vi "ATM.vi"() -> ()   [LabVIEW 2024]
doc: "This VI Simulates the operation of an ATM. It has option to simulate the card, informs the user via the ATM message. It has 6 buttons/ menus that the user can use to select the action he/she wants to perform"
uses:
  Next State.ctl
  Previous State.ctl
  <vilib>/Utility/file.llb/Read Delimited Spreadsheet (string).vi
  <vilib>/Utility/file.llb/Write Delimited Spreadsheet (string).vi
panel:
  in  "Enter":bool
  in  "User Input":string
  in  "Right Buttons\nButtons":T1
  out "Right Menu":T2
  in  "Left Buttons":T1
  out "Left Menu":T2
  in  "Card Simulator":bool
  out "ATM Messages":string
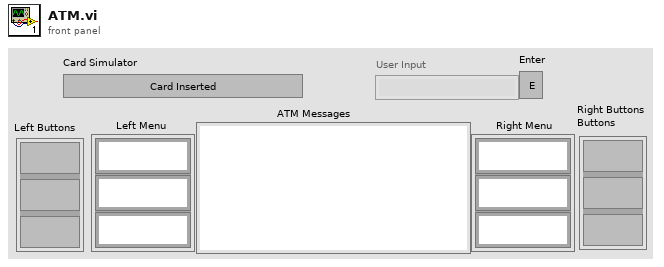
[diagram p1: front panel]
types:
  T1 = cluster{"Func Button":bool, "Func Button 2":bool, "Func Button 3":bool}
  T2 = cluster{"RFS String":string, "RFS String 2":string, "RFS String 3":string}
  T3 = typedef "Previous State.ctl" = enum16{"Start", "Withdraw", "Deposit", "Card Inserted"}
  T4 = cluster{"appended path":path, "Previous State":T3, "User Input":string, "File data":string[][], "Account Number Index":i32}
  T5 = cluster{"User Input":refnum<vi>, "Left Buttons":refnum<vi>, "Right Buttons\nButtons":refnum<vi>, "Enter":refnum<vi>, "Card Simulator":refnum<vi>}
  T6 = typedef "Next State.ctl" = enum16{"Start/Run", "Wait for Event", "Session Terminate", "Exit"}
  T7 = cluster{"Left Menu":cluster{"RFS String":string, "RFS String 2":string, "RFS String 3":string}, "ATM Messages":string, "Right Menu":cluster{"RFS String":string, "RFS String 2":string, "RFS String 3":string}}
  T8 = enum16{"Balance Inquiry", "Withdrawal Failed", "Withdrawal Complete", "Withdrawal", "Deposit Complete", "Deposit", "Session Terminate", "Account Verification Failed", "Main Menu", "Welcome Message"}
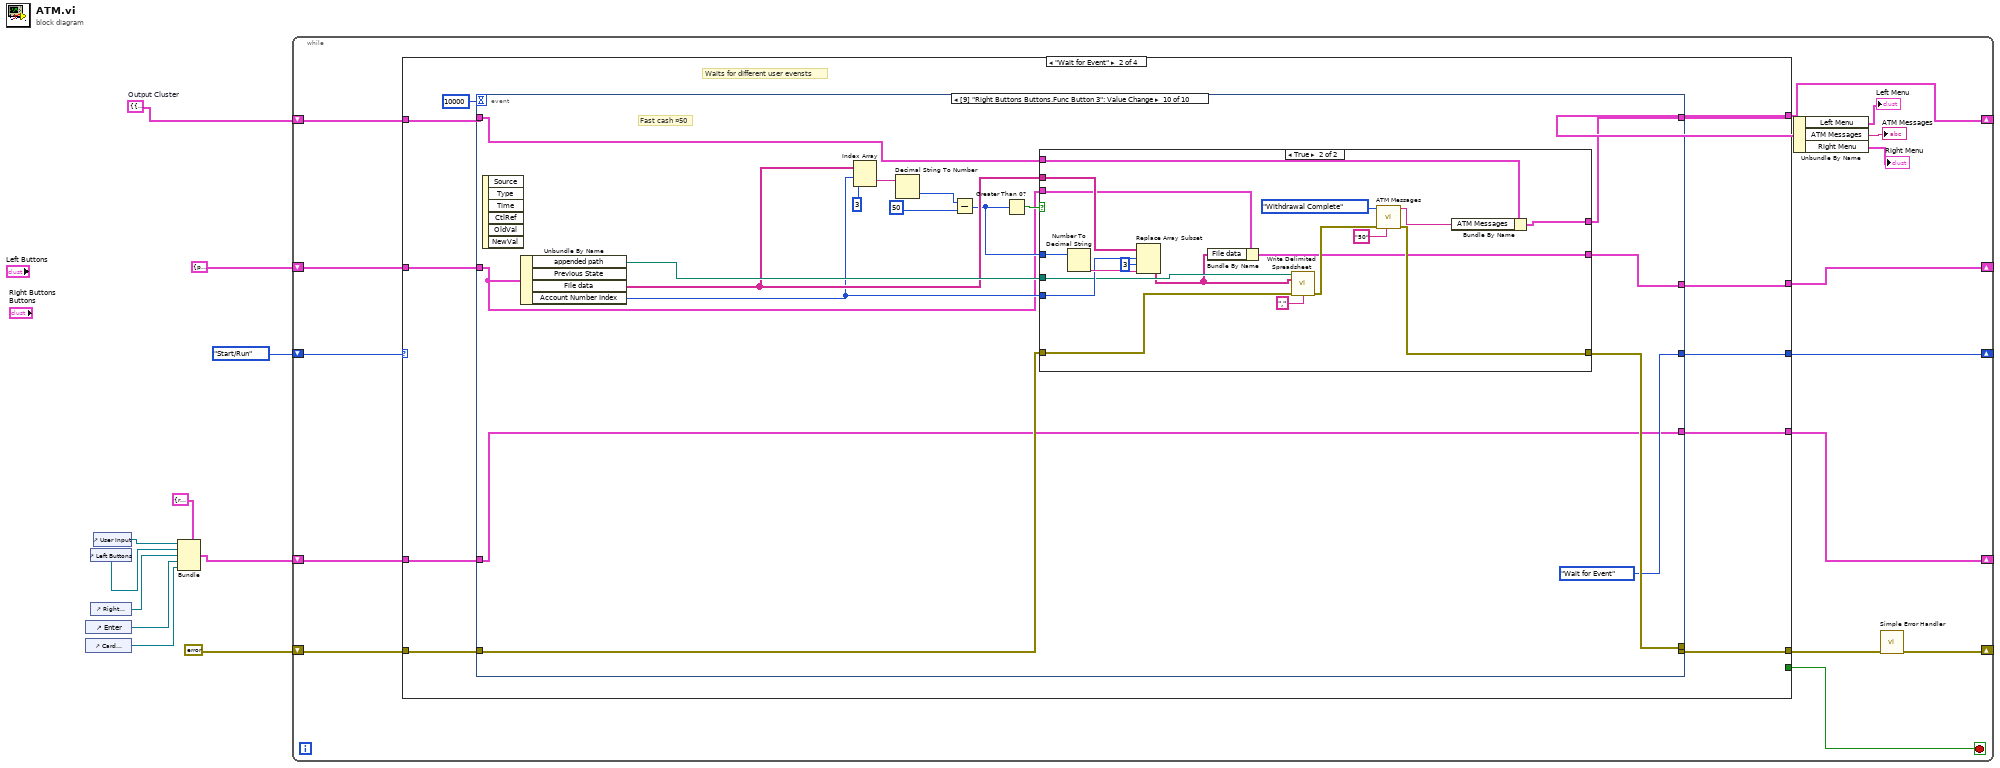
[diagram p0: block diagram]
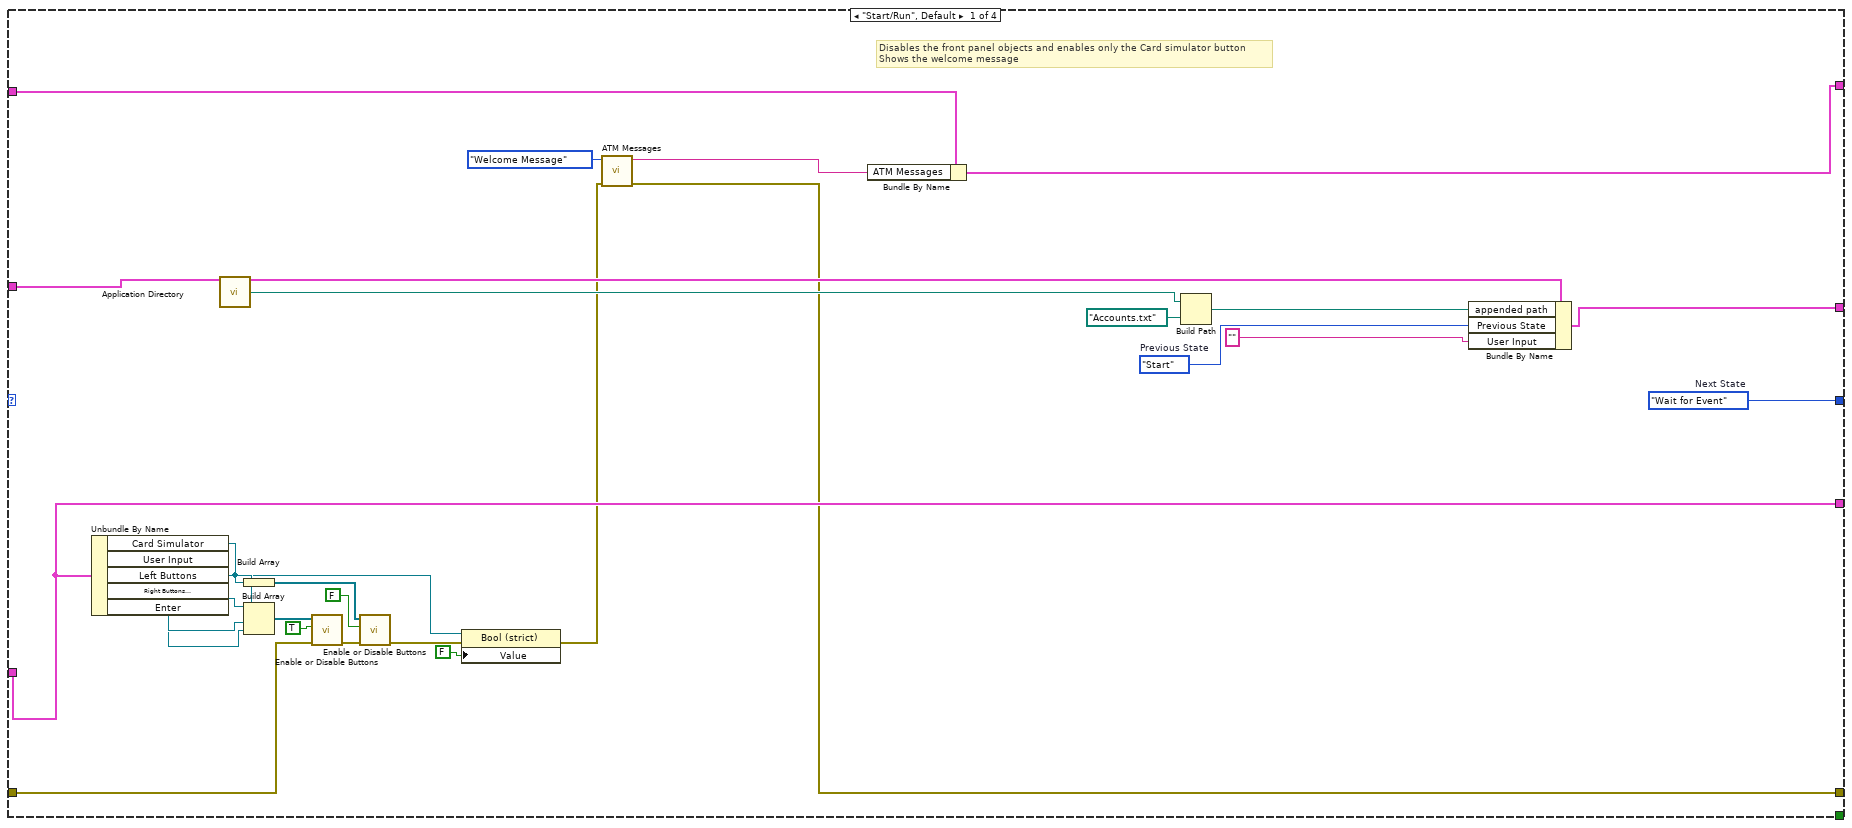
[diagram p2: hidden frame]
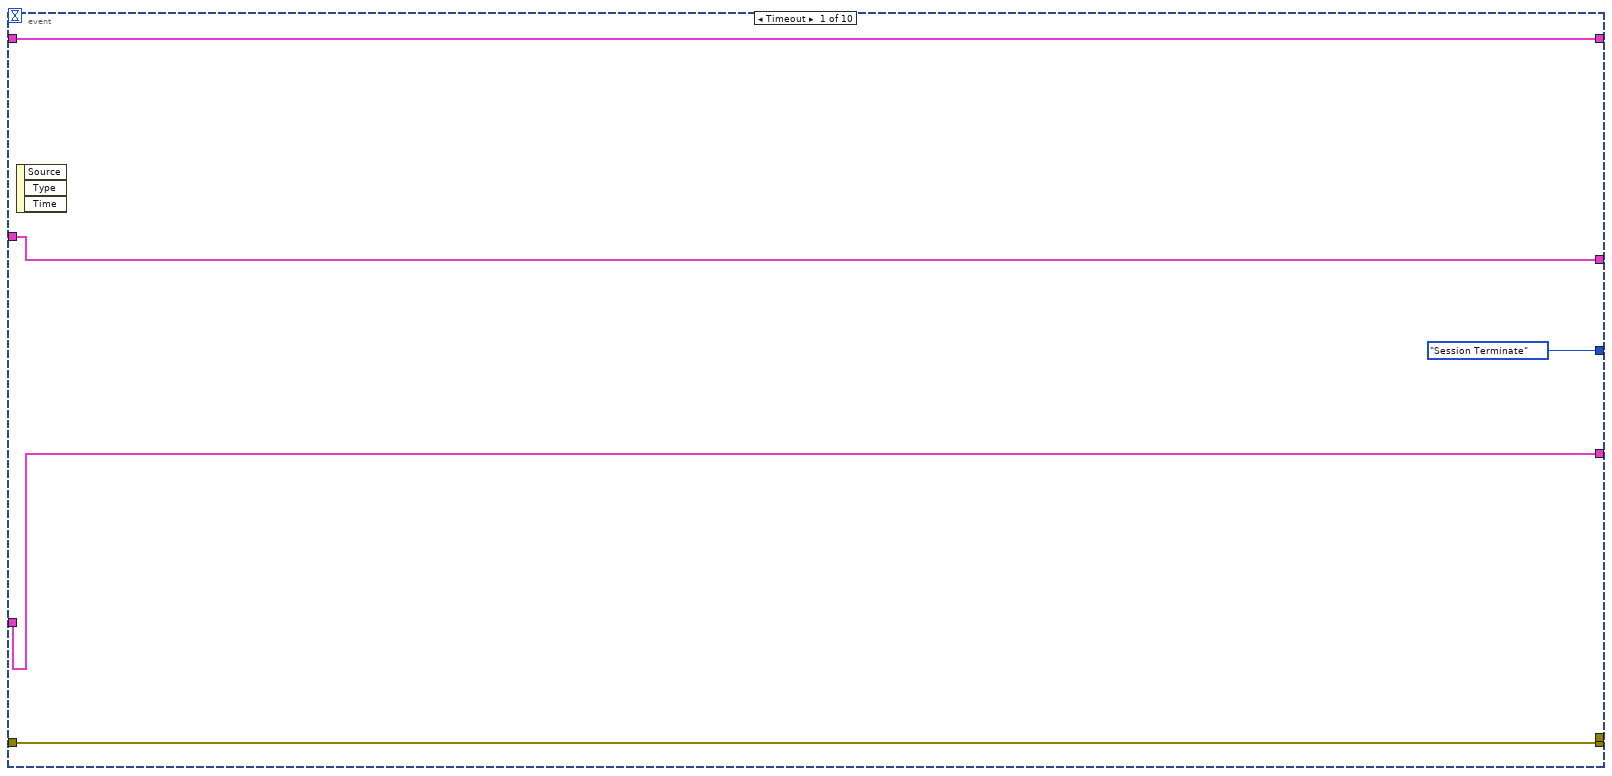
[diagram p3: hidden frame]
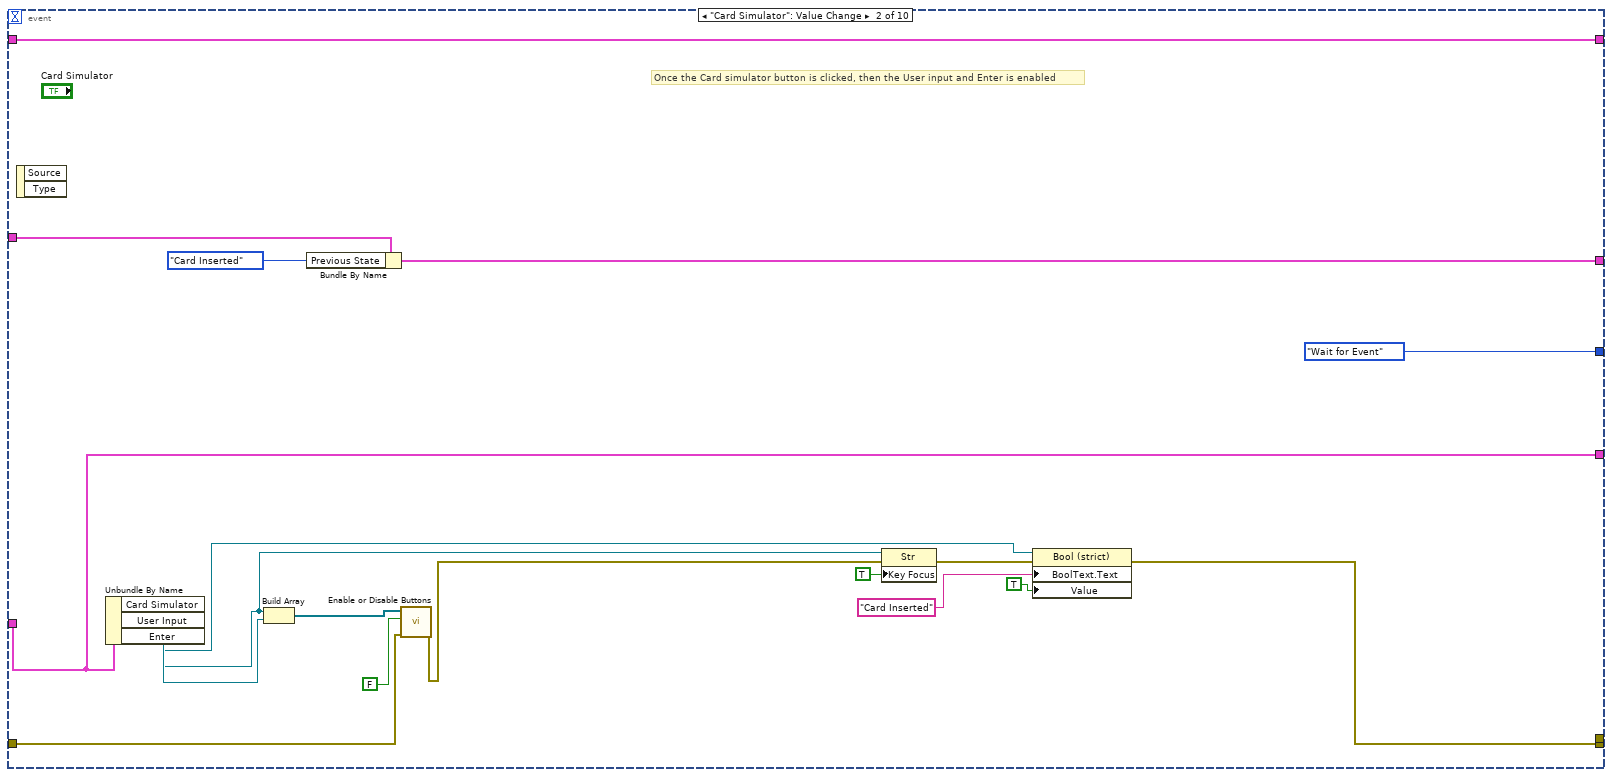
[diagram p4: hidden frame]
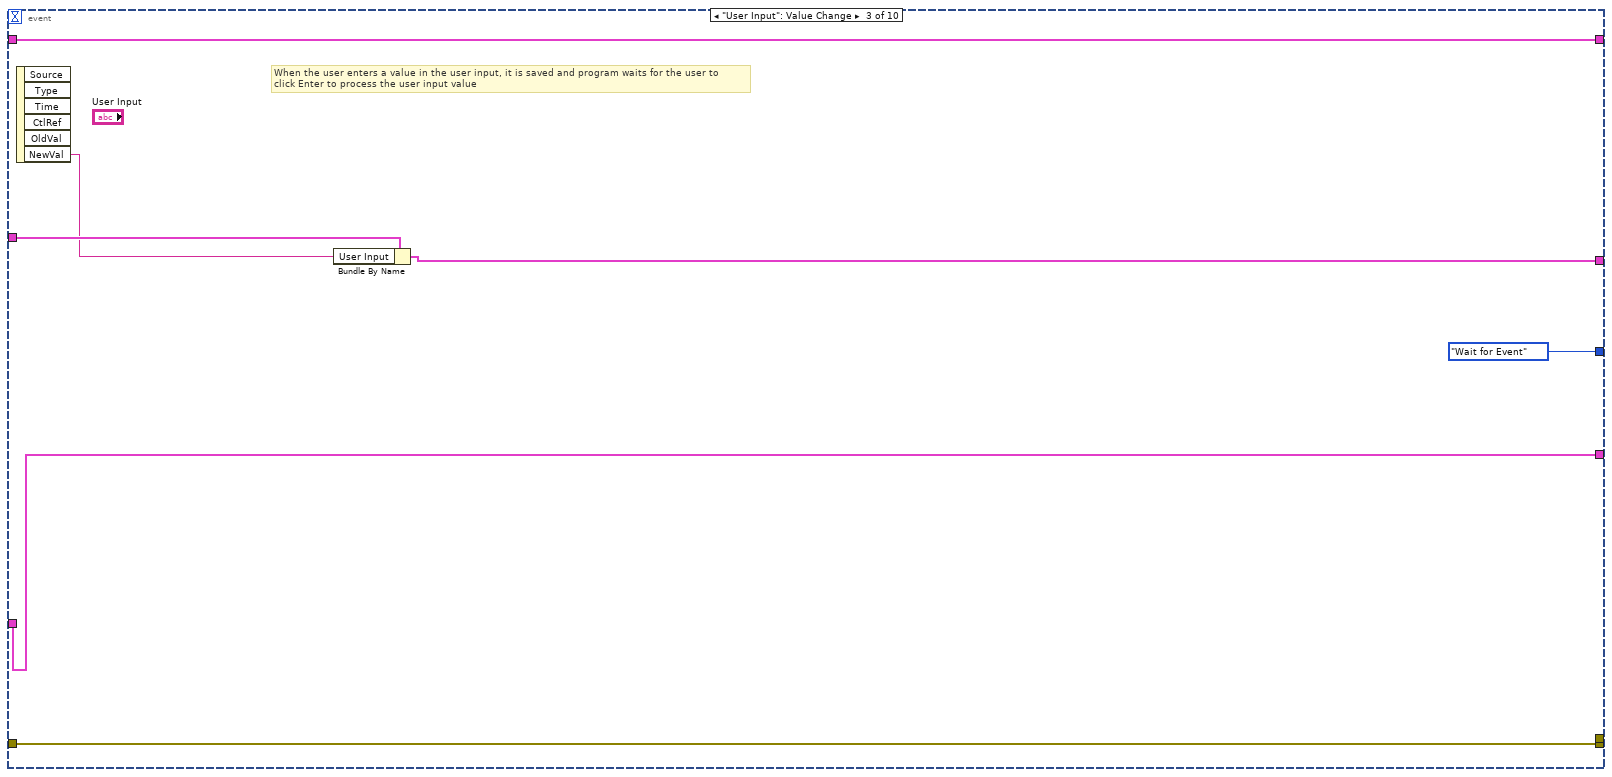
[diagram p5: hidden frame]
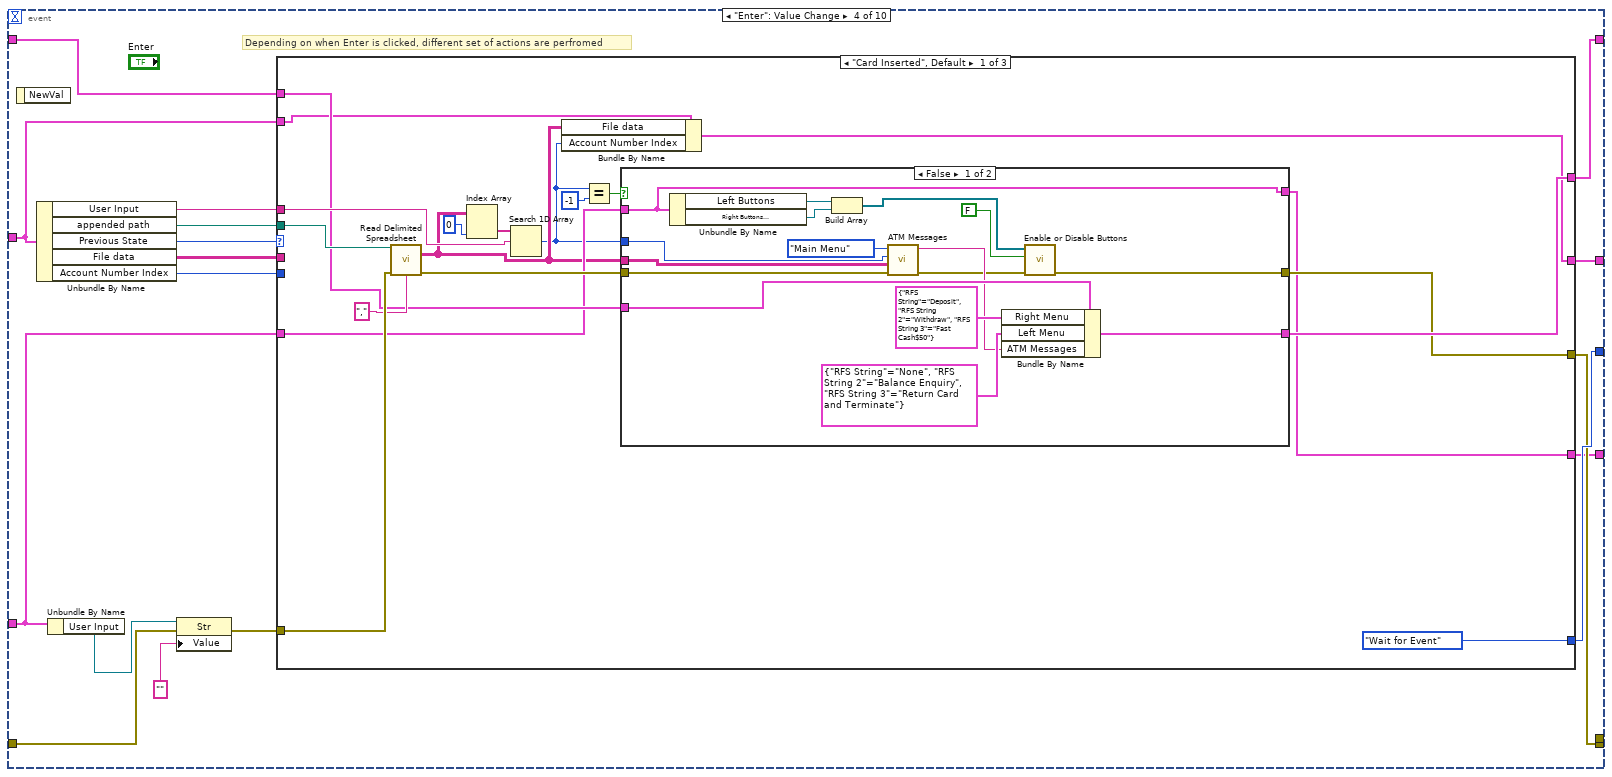
[diagram p6: hidden frame]
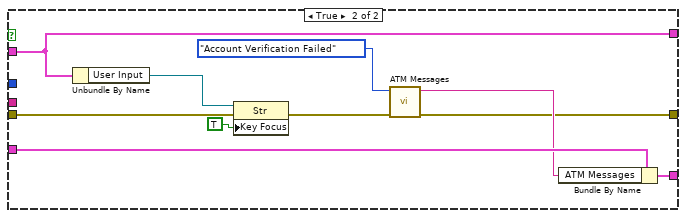
[diagram p7: hidden frame]
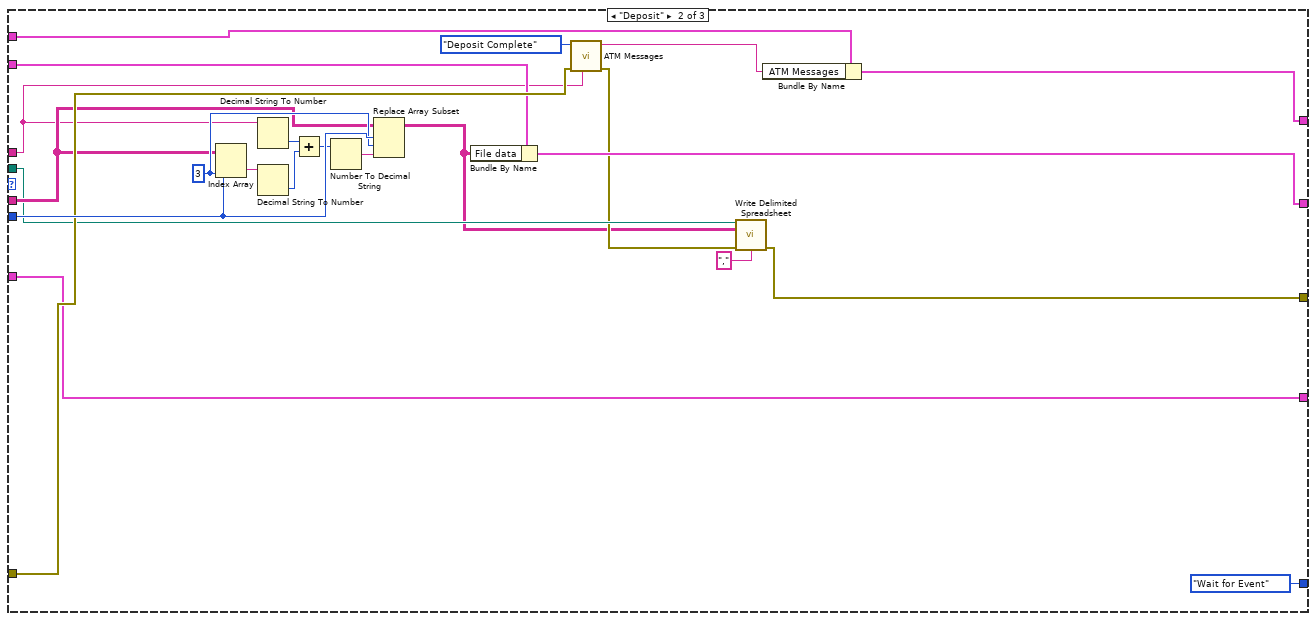
[diagram p8: hidden frame]
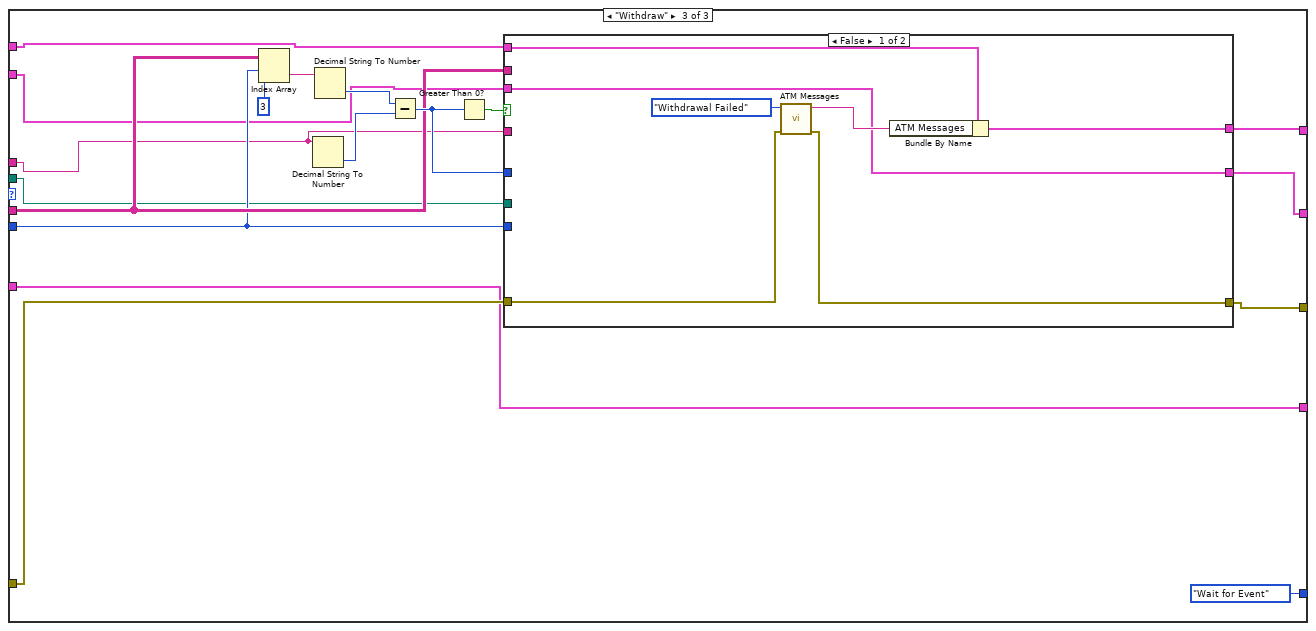
[diagram p9: hidden frame]
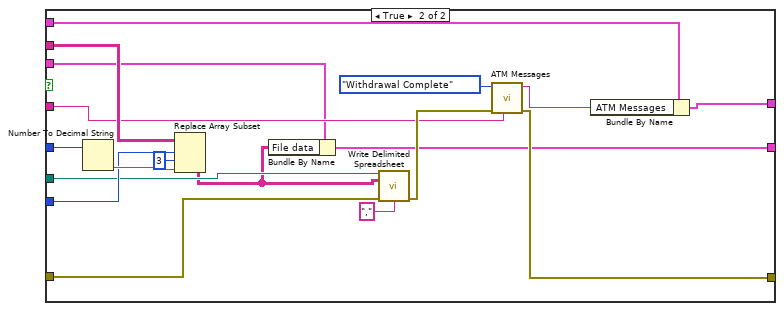
[diagram p10: hidden frame]
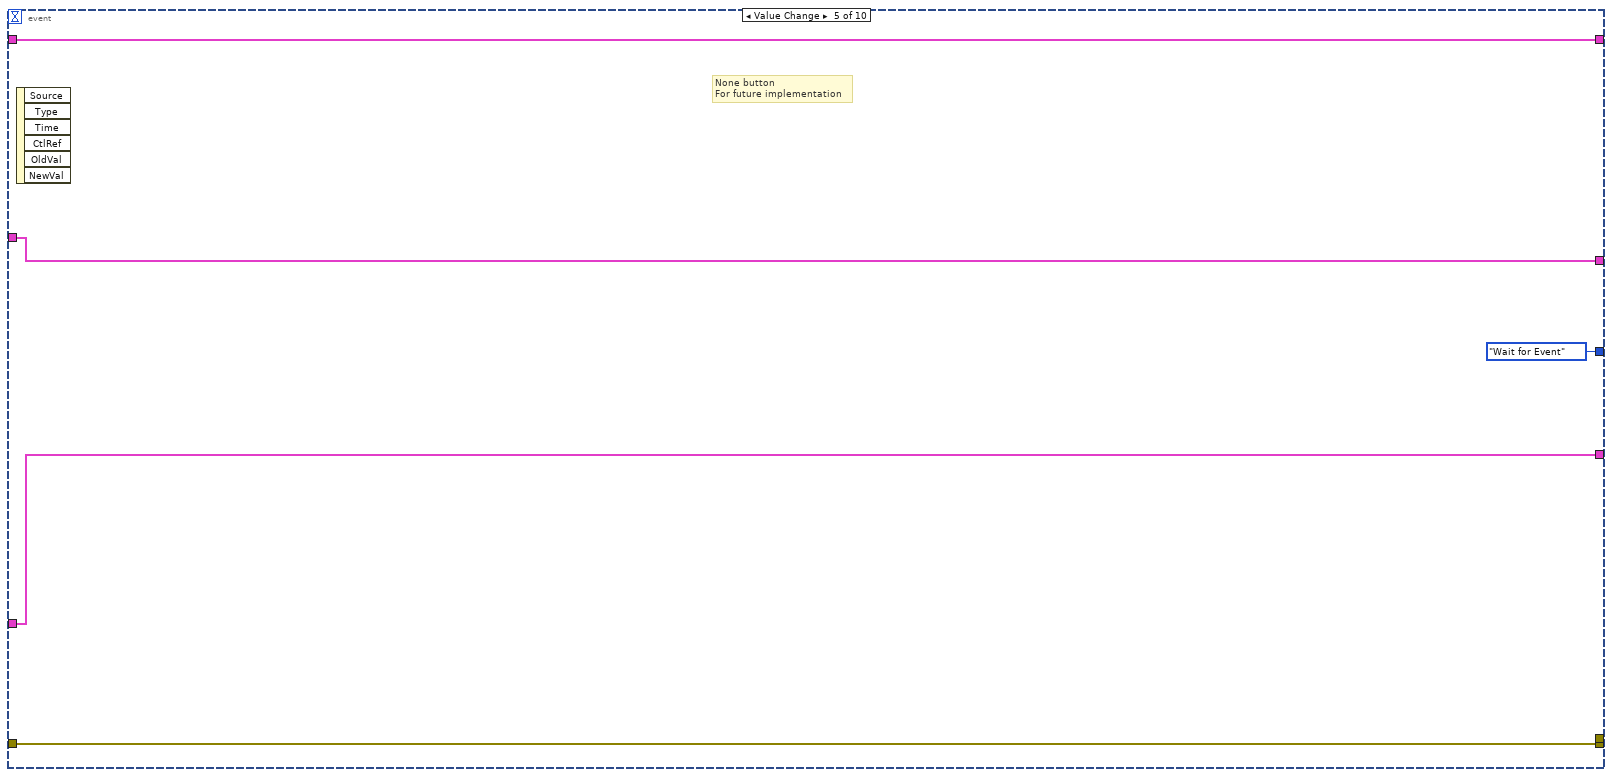
[diagram p11: hidden frame]
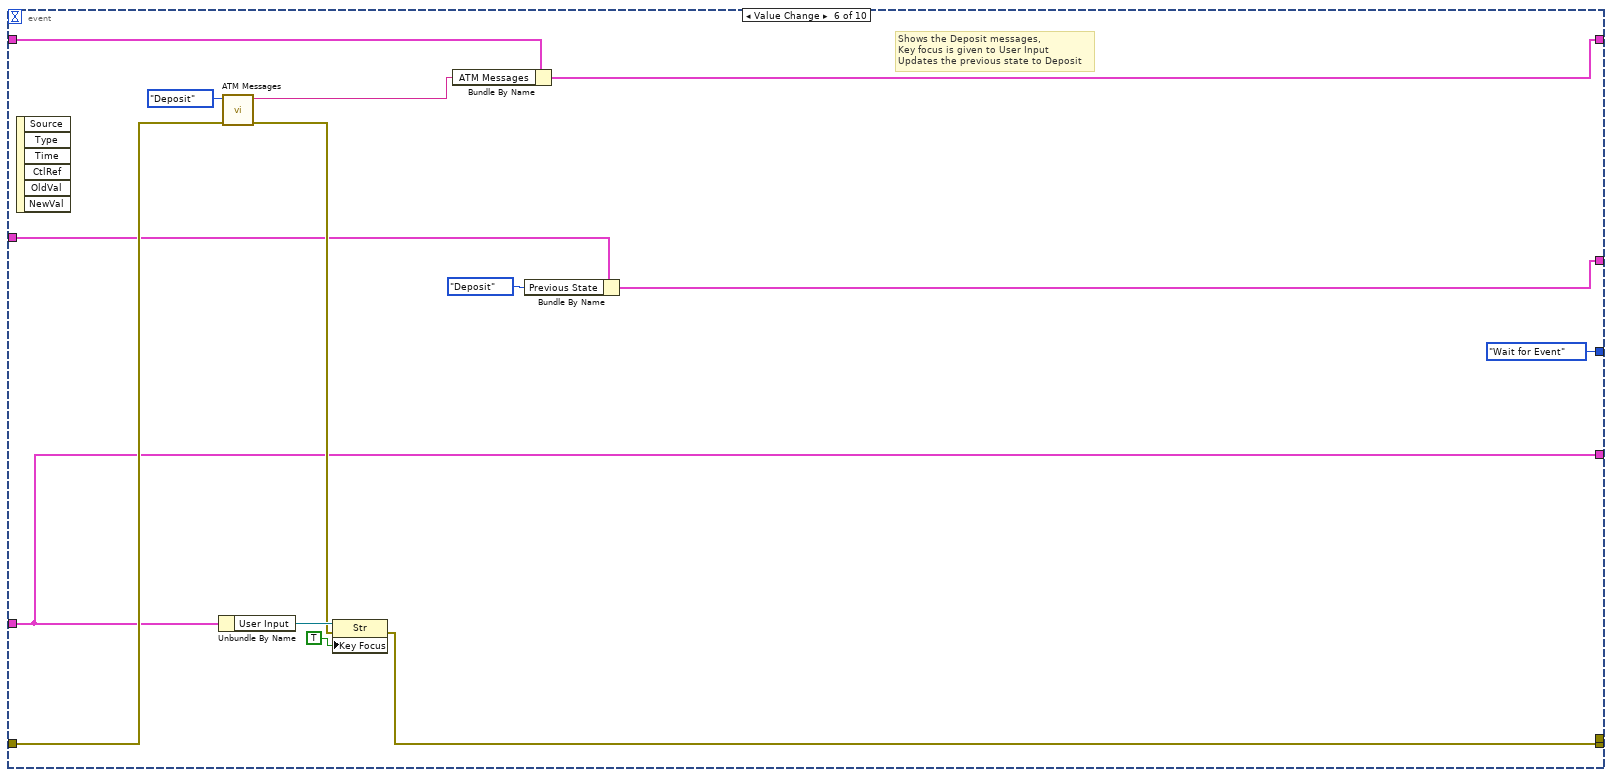
[diagram p12: hidden frame]
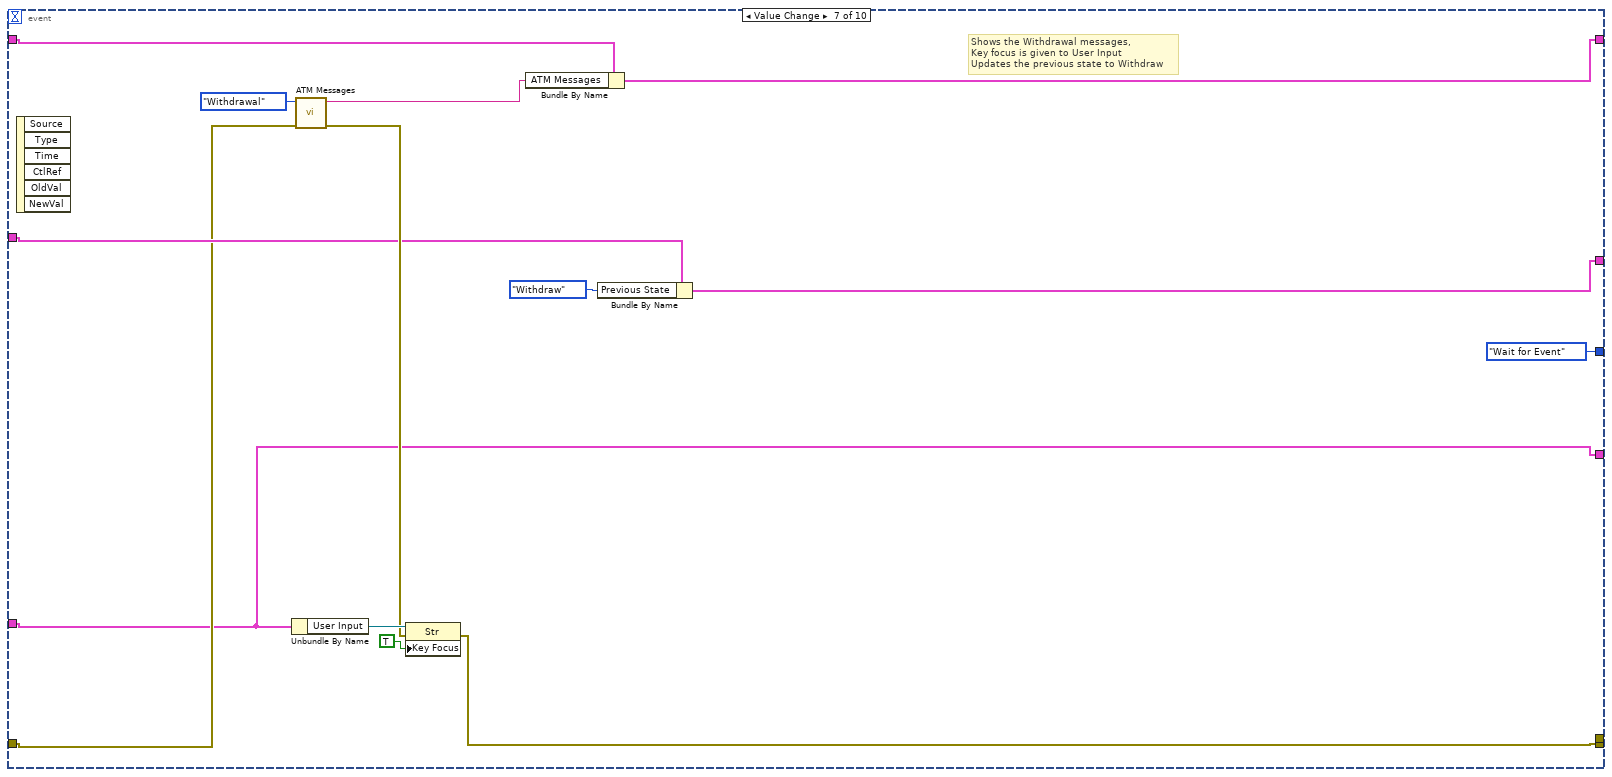
[diagram p13: hidden frame]
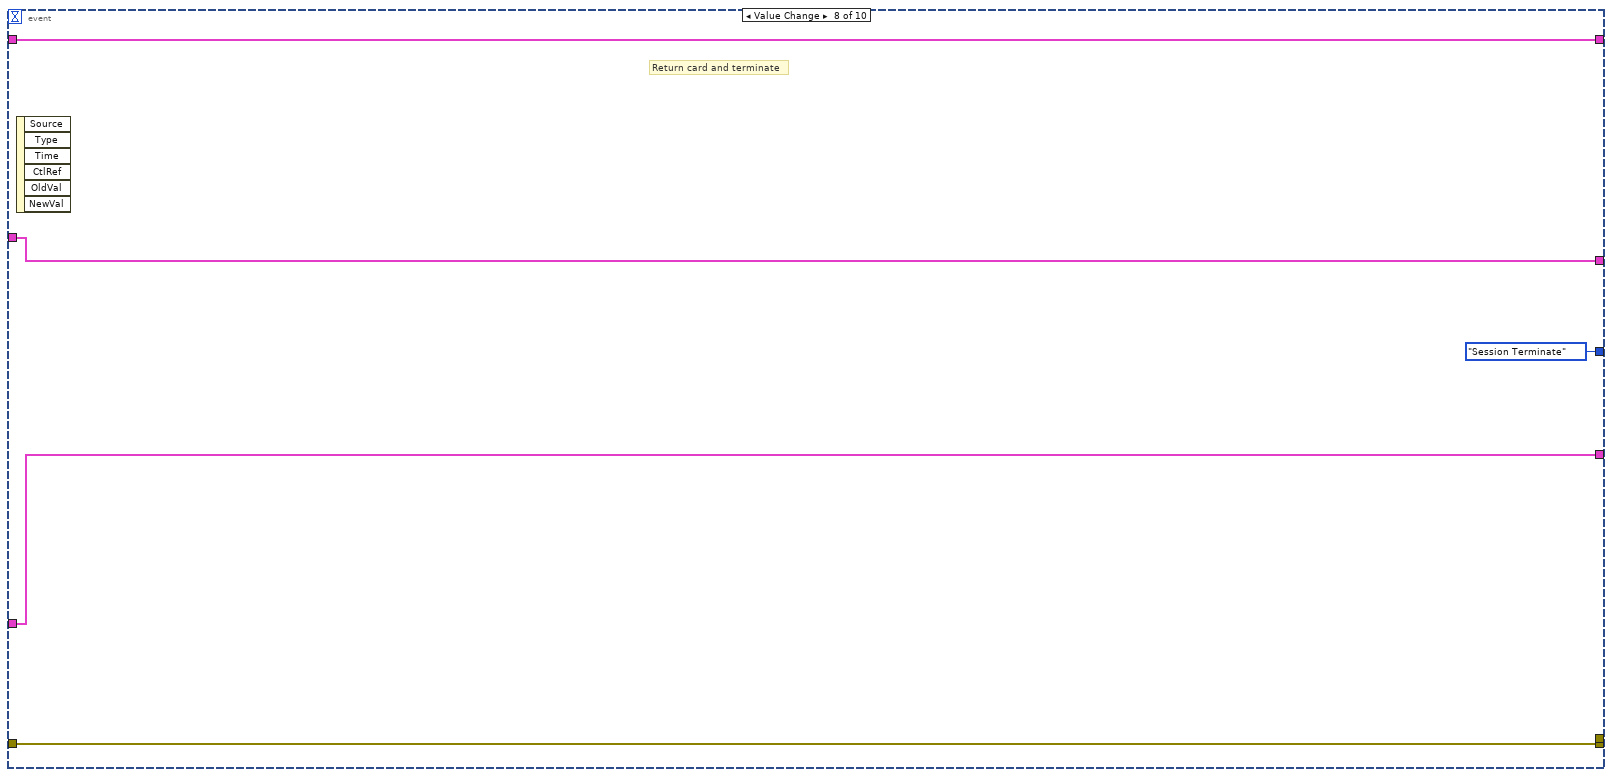
[diagram p14: hidden frame]
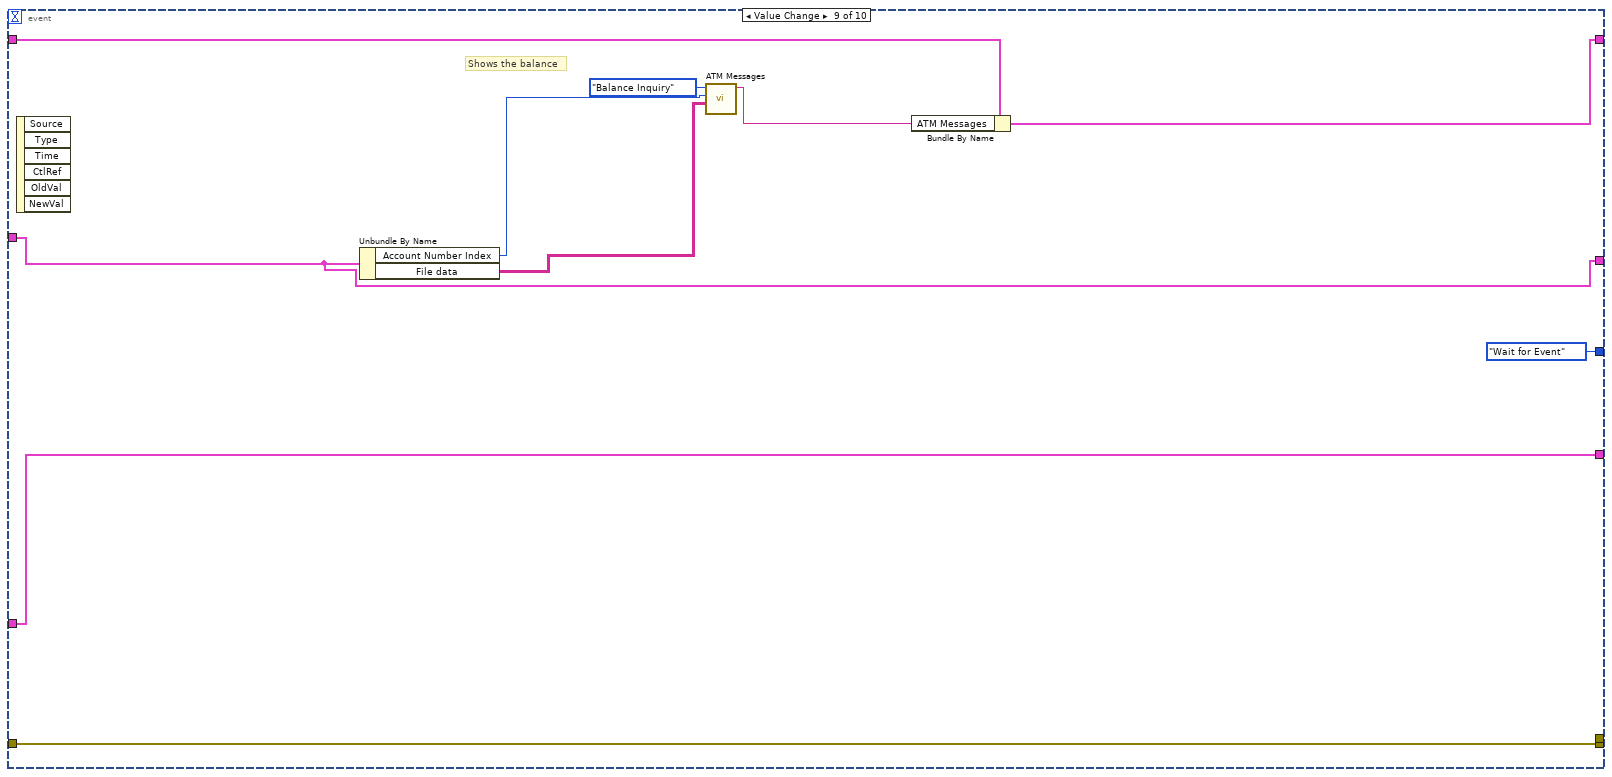
[diagram p15: hidden frame]
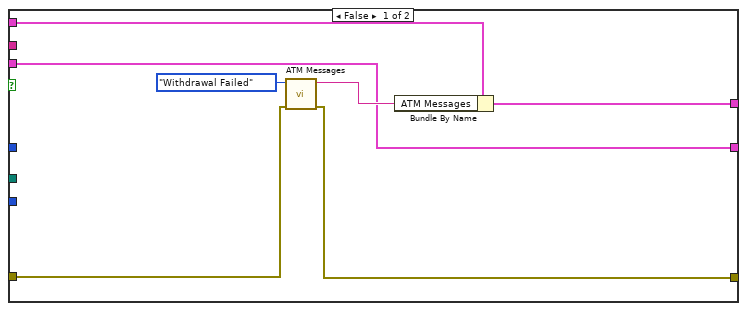
[diagram p16: hidden frame]
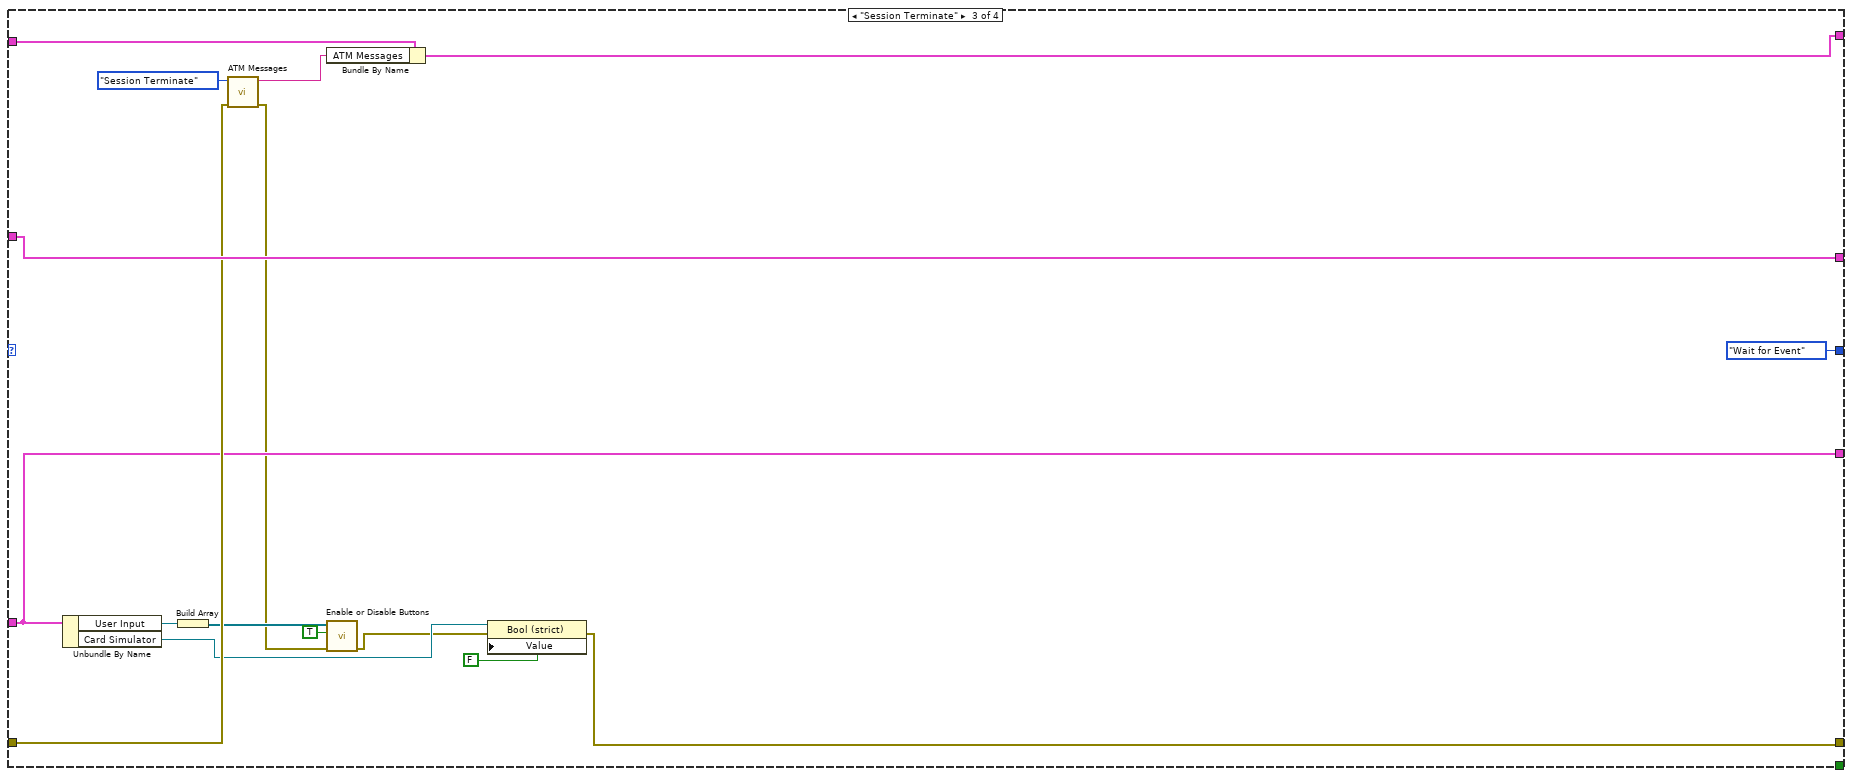
[diagram p17: hidden frame]
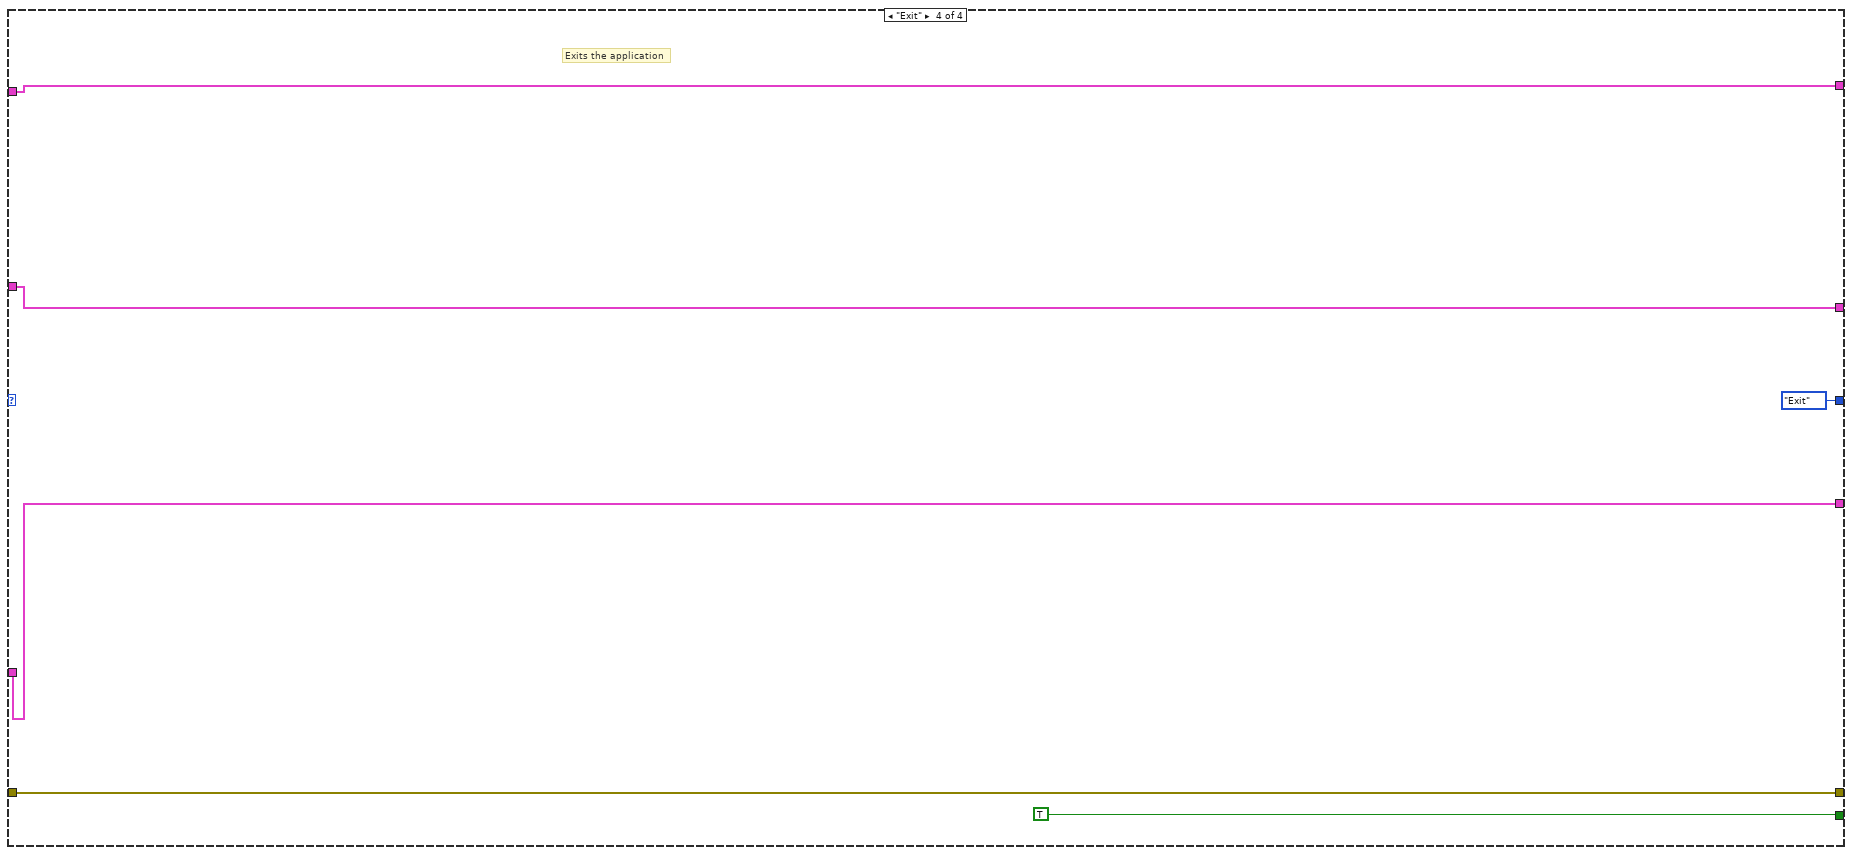
[diagram p18: hidden frame]
diagram:
  w11 = T7 {"Left Menu"={"RFS String"="", "RFS String 2"="", "RFS String 3"=""}, "ATM Messages"="", "Right Menu"={"RFS String"="", "RFS String 2"="", "RFS String 3"=""}}  # Output Cluster
  n1 = control-ref of="Enter"() -> (w6:refnum<vi>)
  n2 = control-ref of="Card Simulator"() -> (w5:refnum<vi>)
  n3 = control-ref of="Left Buttons"() -> (w8:refnum<vi>)
  n4 = control-ref of="Right Buttons\nButtons"() -> (w7:refnum<vi>)
  n5 = control-ref of="User Input"() -> (w9:refnum<vi>)
  n6 = Bundle(cluster=T5 {"User Input"=refnum, "Left Buttons"=refnum, "Right Buttons\nButtons"=refnum, "Enter"=refnum, "Card Simulator"=refnum}, "User Input"=w9, "Left Buttons"=w8, "Right Buttons\nButtons"=w7, "Enter"=w6, "Card Simulator"=w5) -> (w3:T5)
  n7 = while {
    shift-right: [w22] -> _
    shift-left: w11 -> [w26]
    shift-right: [w17] -> _
    shift-left: w3 -> [w19]
    shift-right: [w12] -> _
    shift-left: errorcluster {"status"=FALSE, "code"=0, "source"=""} ("error out") -> [w18]
    shift-right: [w16] -> _
    shift-left: Next_State."Start/Run" -> [w21]
    shift-right: [w14] -> _
    shift-left: T4 {"appended path"=path "", "Previous State"=enum."Withdraw", "User Input"="", "File data"=[], "Account Number Index"=0} ("Data") -> [w15]
    stop <- w20 stop-if-true
    n8 = case shown="\"Wait for Event\"" w21 {
      tunnel: w26 -> [w42 w61 w328 w333]
      tunnel: [w41 w55 w327 w333] -> w22
      tunnel: [_ _ _ TRUE] -> w20
      tunnel: w19 -> [w45 w63 w321 w331]
      tunnel: w18 -> [w48 w62 w322 w329]
      tunnel: [w45 w56 w321 w331] -> w17
      tunnel: [w40 w57 Next_State."Wait for Event" ("Next State") Next_State."Exit" ("Next State")] -> w16
      tunnel: w15 -> [w39 w59 w325 w332]
      tunnel: [w35 w58 w325 w332] -> w14
      tunnel: [w27 w60 w314 w329] -> w13
      frame "Start/Run", Default {
        w40 = Next_State."Wait for Event"  # Next State
        w37 = Previous_State."Start"  # Previous State
        # "Disables the front panel objects and enables only the Card simulator button\nShows the welcome message"
        n9 = Unbundle By Name(w45) -> ("Card Simulator"=w33:refnum<vi>, "User Input"=w54:refnum<vi>, "Left Buttons"=w53:refnum<vi>, "Right Buttons\nButtons"=w52:refnum<vi>, "Enter"=w51:refnum<vi>)
        n10 = call <vilib>:"Application Directory.vi"() -> ("Application Directory"=w44:path)
        n11 = Build Array(w33) -> (w47:refnum<vi>[])
        n12 = Build Array(w54, w53, w52, w51) -> (w50:refnum<vi>[])
        n13 = call "Enable or Disable Buttons.vi"("Error In"=w48, "Disable?"=TRUE, "Refnum array"=w50) -> ("Error Out"=w34:errorcluster)  [unwired: 7 in, 1 out]
        n14 = call "Enable or Disable Buttons.vi"("Error In"=w34, "Disable?"=FALSE, "Refnum array"=w47) -> ("Error Out"=w31:errorcluster)  [unwired: 7 in, 1 out]
        n15 = property class="Bool (strict)"(reference=w33, error in=w31, "Value"=FALSE) -> (error out=w28:errorcluster)  [unwired: 1 out]
        n16 = call "ATM Messages.vi"("Error In"=w28, "Atm Message"=T8."Welcome Message") -> ("error Out"=w27:errorcluster, "ATM Messages"=w29:string)  [unwired: 8 in]
        n17 = Bundle By Name(cluster=w42, "ATM Messages"=w29) -> (w41:T7)
        n18 = Build Path(base path=w44, name or relative path=path "Accounts.txt") -> (appended path=w38:path)
        n19 = Bundle By Name(cluster=w39, "appended path"=w38, "Previous State"=w37, "User Input"="") -> (w35:T4)
      }
      frame "Wait for Event" {
        # "Waits for different user evensts"
        n20 = event shown="[9] \"Right Buttons Buttons.Func Button 3\": Value Change" {
          selector: _ -> [_ _ _ _ _ _ _ _ _ _]
          dyn-events: _ -> [_ _ _ _ _ _ _ _ _ _]
          timeout: 10000 -> [_ _ _ _ _ _ _ _ _ _]
          tunnel: w63 -> [w67 w75 w91 w100 w226 w228 w242 w259 w263 w272]
          tunnel: w62 -> [w66 w84 w92 w110 w227 w235 w247 w260 w264 w278]
          tunnel: w61 -> [w69 w80 w89 w104 w223 w240 w249 w256 w267 w277]
          tunnel: [w69 w80 w89 w103 w223 w238 w243 w256 w265 w271] -> w55
          tunnel: [w66 w71 w92 w101 w227 w233 w246 w260 w264 _] -> w60
          tunnel: w59 -> [w68 w79 w94 w99 w224 w232 w248 w257 w262 w276]
          tunnel: [w68 w77 w93 w97 w224 w230 w244 w257 w262 w275] -> w58
          tunnel: [Next_State."Session Terminate" ("Next State") Next_State."Wait for Event" ("Next State") Next_State."Wait for Event" ("Next State") w105 Next_State."Wait for Event" ("Next State") Next_State."Wait for Event" ("Next State") Next_State."Wait for Event" ("Next State") Next_State."Session Terminate" ("Next State") Next_State."Wait for Event" ("Next State") Next_State."Wait for Event" ("Next State")] -> w57
          tunnel: [w67 w75 w91 w98 w226 w228 w242 w259 w263 w272] -> w56
          tunnel: [_ _ _ _ _ _ _ _ _ w274] -> _
          event Timeout {
            n21 = event-data() -> ()  [unwired: 1 in, 3 out]
          }
          event "Card Simulator": Value Change {
            # "Once the Card simulator button is clicked, then the User input and Enter is enabled"
            n22 = event-data() -> ()  [unwired: 1 in, 2 out]
            n23 = Unbundle By Name(w75) -> ("Card Simulator"=w74:refnum<vi>, "User Input"=w83:refnum<vi>, "Enter"=w87:refnum<vi>)
            n24 = Build Array(w83, w87) -> (w86:refnum<vi>[])
            n25 = Bundle By Name(cluster=w79, "Previous State"=Previous_State."Card Inserted") -> (w77:T4)
            n26 = call "Enable or Disable Buttons.vi"("Error In"=w84, "Disable?"=FALSE, "Refnum array"=w86) -> ("Error Out"=w82:errorcluster)  [unwired: 7 in, 1 out]
            n27 = property class="Str"(reference=w83, error in=w82, "Key Focus"=TRUE) -> (error out=w72:errorcluster)  [unwired: 1 out]
            n28 = property class="Bool (strict)"(reference=w74, error in=w72, "BoolText.Text"="Card Inserted" ("Boolean Text.Text"), "Value"=TRUE) -> (error out=w71:errorcluster)  [unwired: 1 out]
          }
          event "User Input": Value Change {
            # "When the user enters a value in the user input, it is saved and program waits for the user to \nclick Enter to process the user input value"
            n29 = event-data() -> ("NewVal"=w88:string)  [unwired: 1 in, 5 out]
            n30 = Bundle By Name(cluster=w94, "User Input"=w88) -> (w93:T4)
          }
          event "Enter": Value Change {
            # "Depending on when Enter is clicked, different set of actions are perfromed"
            n31 = event-data() -> ()  [unwired: 1 in, 1 out]
            n32 = Unbundle By Name(w99) -> ("User Input"=w107:string, "appended path"=w108:path, "Previous State"=w111:T3, "File data"=w96:string[][], "Account Number Index"=w95:i32)
            n33 = Unbundle By Name(w100) -> ("User Input"=w102:refnum<vi>)
            n34 = property class="Str"(reference=w102, error in=w110, "Value"="") -> (error out=w106:errorcluster)  [unwired: 1 out]
            n35 = case shown="\"Card Inserted\", Default" w111 {
              tunnel: w108 -> [w130 w161 w187]
              tunnel: w107 -> [w125 w162 w186]
              tunnel: w106 -> [w129 w172 w191]
              tunnel: [Next_State."Wait for Event" ("Next State") Next_State."Wait for Event" ("Next State") Next_State."Wait for Event" ("Next State")] -> w105
              tunnel: w104 -> [w122 w170 w192]
              tunnel: [w121 w168 w184] -> w103
              tunnel: [w119 w159 w185] -> w101
              tunnel: w100 -> [w118 w167 w183]
              tunnel: w99 -> [w117 w165 w181]
              tunnel: [w116 w167 w183] -> w98
              tunnel: [w115 w164 w180] -> w97
              tunnel: w96 -> [_ w163 w189]
              tunnel: w95 -> [_ w176 w188]
              frame "Card Inserted", Default {
                n36 = call-poly <vilib>:"Read Delimited Spreadsheet.vi"("file path (dialog if empty)"=w130, "error in (no error)"=w129, "delimiter (\\t)"="," ("delimiter (\\t)")) -> ("all rows"=w113:string[][], "error out"=w120:errorcluster)  [unwired: 7 in, 4 out]
                n37 = Index Array(array=w113, index (col)=0 ("disabled index (col)")) -> (element=w114:string[])  [unwired: 1 in]
                n38 = Search 1D Array(1D array=w114, element=w125) -> (index of element=w112:i32)  [unwired: 1 in]
                n39 = Bundle By Name(cluster=w117, "File data"=w113, "Account Number Index"=w112) -> (w115:T4)
                n40 = Equal?(x=w112, y=-1) -> (x = y?=w123:bool)
                n41 = case shown="False" w123 {
                  tunnel: w122 -> [w141 w156]
                  tunnel: [w132 w155] -> w121
                  tunnel: w120 -> [w137 w154]
                  tunnel: [w142 w149] -> w119
                  tunnel: w112 -> [w133 _]
                  tunnel: w118 -> [w131 w147]
                  tunnel: w113 -> [w134 _]
                  tunnel: [w131 w147] -> w116
                  frame False {
                    n42 = Unbundle By Name(w131) -> ("Left Buttons"=w146:refnum<vi>, "Right Buttons\nButtons"=w145:refnum<vi>)
                    n43 = Build Array(w146, w145) -> (w144:refnum<vi>[])
                    n44 = call "ATM Messages.vi"("Error In"=w137, "File Data"=w134, "Index of Acount"=w133, "Atm Message"=T8."Main Menu") -> ("error Out"=w136:errorcluster, "ATM Messages"=w138:string)  [unwired: 6 in]
                    n45 = Bundle By Name(cluster=w141, "Right Menu"=T2 {"RFS String"="Deposit", "RFS String 2"="Withdraw", "RFS String 3"="Fast Cash$50"} ("Left Menu"), "Left Menu"=T2 {"RFS String"="None", "RFS String 2"="Balance Enquiry", "RFS String 3"="Return Card and Terminate"} ("Right Menu"), "ATM Messages"=w138) -> (w132:T7)
                    n46 = call "Enable or Disable Buttons.vi"("Error In"=w136, "Disable?"=FALSE, "Refnum array"=w144) -> ("Error Out"=w142:errorcluster)  [unwired: 7 in, 1 out]
                  }
                  frame True {
                    n47 = Unbundle By Name(w147) -> ("User Input"=w152:refnum<vi>)
                    n48 = property class="Str"(reference=w152, error in=w154, "Key Focus"=TRUE) -> (error out=w150:errorcluster)  [unwired: 1 out]
                    n49 = call "ATM Messages.vi"("Error In"=w150, "Atm Message"=T8."Account Verification Failed") -> ("error Out"=w149:errorcluster, "ATM Messages"=w151:string)  [unwired: 8 in]
                    n50 = Bundle By Name(cluster=w156, "ATM Messages"=w151) -> (w155:T7)
                  }
                }
              }
              frame "Deposit" {
                w175 = 3 ("disabled index (col)")
                n51 = Index Array(array=w163, index (row)=w176, index (col)=w175) -> (element=w179:string)
                n52 = Decimal String To Number(string=w162) -> (number=w178:i32)  [unwired: 2 in, 1 out]
                n53 = Decimal String To Number(string=w179) -> (number=w177:i32)  [unwired: 2 in, 1 out]
                n54 = Add(x=w178, y=w177) -> (x+y=w174:i32)
                n55 = Number To Decimal String(number=w174) -> (decimal integer string=w173:string)  [unwired: 1 in]
                n56 = Replace Array Subset(array=w163, new element=w173, index (row)=w176, index (col)=w175) -> (w158:string[][])
                n57 = Bundle By Name(cluster=w165, "File data"=w158) -> (w164:T4)
                n58 = call "ATM Messages.vi"("User Input"=w162, "Error In"=w172, "Atm Message"=T8."Deposit Complete") -> ("error Out"=w160:errorcluster, "ATM Messages"=w169:string)  [unwired: 7 in]
                n59 = call-poly <vilib>:"Write Delimited Spreadsheet.vi"("file path (dialog if empty)"=w161, "2D data"=w158, "error in (no error)"=w160, "delimiter (\\t)"="," ("delimiter (\\t)")) -> ("error out"=w159:errorcluster)  [unwired: 10 in, 1 out]
                n60 = Bundle By Name(cluster=w170, "ATM Messages"=w169) -> (w168:T7)
              }
              frame "Withdraw" {
                n61 = Index Array(array=w189, index (row)=w188, index (col)=3 ("disabled index (col)")) -> (element=w194:string)
                n62 = Decimal String To Number(string=w186) -> (number=w196:i32)  [unwired: 2 in, 1 out]
                n63 = Decimal String To Number(string=w194) -> (number=w197:i32)  [unwired: 2 in, 1 out]
                n64 = Subtract(x=w197, y=w196) -> (x-y=w190:i32)
                n65 = Greater Than 0?(x=w190) -> (x > 0?=w193:bool)
                n66 = case shown="False" w193 {
                  tunnel: w192 -> [w201 w221]
                  tunnel: w191 -> [w203 w208]
                  tunnel: [w202 w218] -> w185
                  tunnel: [w199 w219] -> w184
                  tunnel: w190 -> [_ w217]
                  tunnel: w189 -> [_ w215]
                  tunnel: w188 -> [_ w214]
                  tunnel: w187 -> [_ w211]
                  tunnel: w186 -> [_ w209]
                  tunnel: w181 -> [w198 w207]
                  tunnel: [w198 w205] -> w180
                  frame False {
                    n67 = call "ATM Messages.vi"("Error In"=w203, "Atm Message"=T8."Withdrawal Failed") -> ("error Out"=w202:errorcluster, "ATM Messages"=w200:string)  [unwired: 8 in]
                    n68 = Bundle By Name(cluster=w201, "ATM Messages"=w200) -> (w199:T7)
                  }
                  frame True {
                    n69 = Number To Decimal String(number=w217) -> (decimal integer string=w216:string)  [unwired: 1 in]
                    n70 = Replace Array Subset(array=w215, new element=w216, index (row)=w214, index (col)=3 ("disabled index (col)")) -> (w206:string[][])
                    n71 = Bundle By Name(cluster=w207, "File data"=w206) -> (w205:T4)
                    n72 = call-poly <vilib>:"Write Delimited Spreadsheet.vi"("file path (dialog if empty)"=w211, "2D data"=w206, "error in (no error)"=w208, "delimiter (\\t)"="," ("delimiter (\\t)")) -> ("error out"=w210:errorcluster)  [unwired: 10 in, 1 out]
                    n73 = call "ATM Messages.vi"("User Input"=w209, "Error In"=w210, "Atm Message"=T8."Withdrawal Complete") -> ("error Out"=w218:errorcluster, "ATM Messages"=w220:string)  [unwired: 7 in]
                    n74 = Bundle By Name(cluster=w221, "ATM Messages"=w220) -> (w219:T7)
                  }
                }
              }
            }
          }
          event "Left Buttons.Func Button": Value Change {
            # "None button\nFor future implementation"
            n75 = event-data() -> ()  [unwired: 1 in, 6 out]
          }
          event "Right Buttons\nButtons.Func Button": Value Change {
            # "Shows the Deposit messages,  \nKey focus is given to User Input\nUpdates the previous state to Deposit"
            n76 = event-data() -> ()  [unwired: 1 in, 6 out]
            n77 = Unbundle By Name(w228) -> ("User Input"=w237:refnum<vi>)
            n78 = call "ATM Messages.vi"("Error In"=w235, "Atm Message"=T8."Deposit") -> ("error Out"=w234:errorcluster, "ATM Messages"=w239:string)  [unwired: 8 in]
            n79 = property class="Str"(reference=w237, error in=w234, "Key Focus"=TRUE) -> (error out=w233:errorcluster)  [unwired: 1 out]
            n80 = Bundle By Name(cluster=w240, "ATM Messages"=w239) -> (w238:T7)
            n81 = Bundle By Name(cluster=w232, "Previous State"=Previous_State."Deposit") -> (w230:T4)
          }
          event "Right Buttons\nButtons.Func Button 2": Value Change {
            # "Shows the Withdrawal messages,  \nKey focus is given to User Input\nUpdates the previous state to Withdraw"
            n82 = event-data() -> ()  [unwired: 1 in, 6 out]
            n83 = Unbundle By Name(w242) -> ("User Input"=w253:refnum<vi>)
            n84 = call "ATM Messages.vi"("Error In"=w247, "Atm Message"=T8."Withdrawal") -> ("error Out"=w251:errorcluster, "ATM Messages"=w254:string)  [unwired: 8 in]
            n85 = property class="Str"(reference=w253, error in=w251, "Key Focus"=TRUE) -> (error out=w246:errorcluster)  [unwired: 1 out]
            n86 = Bundle By Name(cluster=w249, "ATM Messages"=w254) -> (w243:T7)
            n87 = Bundle By Name(cluster=w248, "Previous State"=Previous_State."Withdraw") -> (w244:T4)
          }
          event "Left Buttons.Func Button 3": Value Change {
            # "Return card and terminate"
            n88 = event-data() -> ()  [unwired: 1 in, 6 out]
          }
          event "Left Buttons.Func Button 2": Value Change {
            # "Shows the balance"
            n89 = event-data() -> ()  [unwired: 1 in, 6 out]
            n90 = Unbundle By Name(w262) -> ("Account Number Index"=w268:i32, "File data"=w269:string[][])
            n91 = call "ATM Messages.vi"("File Data"=w269, "Index of Acount"=w268, "Atm Message"=T8."Balance Inquiry") -> ("ATM Messages"=w266:string)  [unwired: 7 in, 1 out]
            n92 = Bundle By Name(cluster=w267, "ATM Messages"=w266) -> (w265:T7)
          }
          event "Right Buttons\nButtons.Func Button 3": Value Change {
            # "Fast cash ¤50"
            n93 = event-data() -> ()  [unwired: 1 in, 6 out]
            n94 = Unbundle By Name(w276) -> ("appended path"=w287:path, "File data"=w286:string[][], "Account Number Index"=w285:i32)  [unwired: 1 out]
            n95 = Index Array(array=w286, index (row)=w285, index (col)=3 ("disabled index (col)")) -> (element=w282:string)
            n96 = Decimal String To Number(string=w282) -> (number=w284:i32)  [unwired: 2 in, 1 out]
            n97 = Subtract(x=w284, y=50) -> (x-y=w280:i32)
            n98 = Greater Than 0?(x=w280) -> (x > 0?=w281:bool)
            n99 = case shown="True" w281 {
              tunnel: w277 -> [w291 w311]
              tunnel: w278 -> [w293 w299]
              tunnel: [w292 w308] -> w274
              tunnel: [w289 w309] -> w271
              tunnel: w280 -> [_ w307]
              tunnel: w286 -> [_ w305]
              tunnel: w285 -> [_ w304]
              tunnel: w287 -> [_ w301]
              tunnel: w276 -> [w288 w298]
              tunnel: [w288 w296] -> w275
              frame False {
                n100 = call "ATM Messages.vi"("Error In"=w293, "Atm Message"=T8."Withdrawal Failed") -> ("error Out"=w292:errorcluster, "ATM Messages"=w290:string)  [unwired: 8 in]
                n101 = Bundle By Name(cluster=w291, "ATM Messages"=w290) -> (w289:T7)
              }
              frame True {
                n102 = Number To Decimal String(number=w307) -> (decimal integer string=w306:string)  [unwired: 1 in]
                n103 = Replace Array Subset(array=w305, new element=w306, index (row)=w304, index (col)=3 ("disabled index (col)")) -> (w297:string[][])
                n104 = Bundle By Name(cluster=w298, "File data"=w297) -> (w296:T4)
                n105 = call-poly <vilib>:"Write Delimited Spreadsheet.vi"("file path (dialog if empty)"=w301, "2D data"=w297, "error in (no error)"=w299, "delimiter (\\t)"="," ("delimiter (\\t)")) -> ("error out"=w300:errorcluster)  [unwired: 10 in, 1 out]
                n106 = call "ATM Messages.vi"("User Input"="50", "Error In"=w300, "Atm Message"=T8."Withdrawal Complete") -> ("error Out"=w308:errorcluster, "ATM Messages"=w310:string)  [unwired: 7 in]
                n107 = Bundle By Name(cluster=w311, "ATM Messages"=w310) -> (w309:T7)
              }
            }
          }
        }
      }
      frame "Session Terminate" {
        n108 = Unbundle By Name(w321) -> ("User Input"=w320:refnum<vi>, "Card Simulator"=w316:refnum<vi>)
        n109 = Build Array(w320) -> (w319:refnum<vi>[])
        n110 = call "ATM Messages.vi"("Error In"=w322, "Atm Message"=T8."Session Terminate") -> ("error Out"=w318:errorcluster, "ATM Messages"=w323:string)  [unwired: 8 in]
        n111 = Bundle By Name(cluster=w328, "ATM Messages"=w323) -> (w327:T7)
        n112 = call "Enable or Disable Buttons.vi"("Error In"=w318, "Disable?"=TRUE, "Refnum array"=w319) -> ("Error Out"=w315:errorcluster)  [unwired: 7 in, 1 out]
        n113 = property class="Bool (strict)"(reference=w316, error in=w315, "Value"=FALSE) -> (error out=w314:errorcluster)  [unwired: 1 out]
      }
      frame "Exit" {
        # "Exits the application"
      }
    }
    n114 = Unbundle By Name(w22) -> ("Left Menu"=→"Left Menu":T2, "ATM Messages"=→"ATM Messages":string, "Right Menu"=→"Right Menu":T2)
    n115 = call <vilib>:"Simple Error Handler.vi"("error in (no error)"=w13) -> ("error out"=w12:errorcluster)  [unwired: 4 in, 4 out]
  }
